vi "random number array generator.vi"() -> ()   [LabVIEW 2015]
panel:
  out "Random Numbers":dbl[](graph)
  in  "Iterations":i32
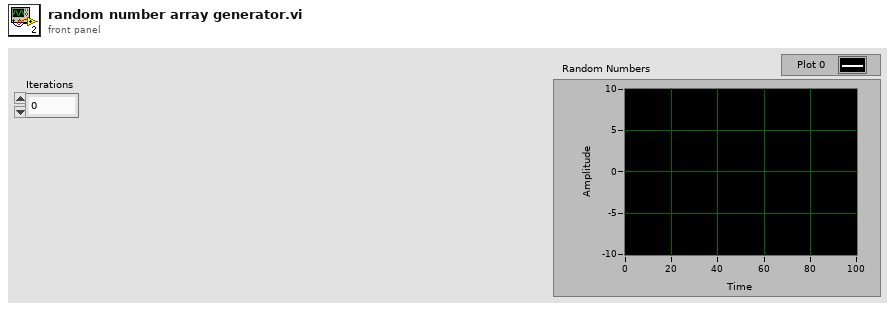
[diagram p1: front panel]
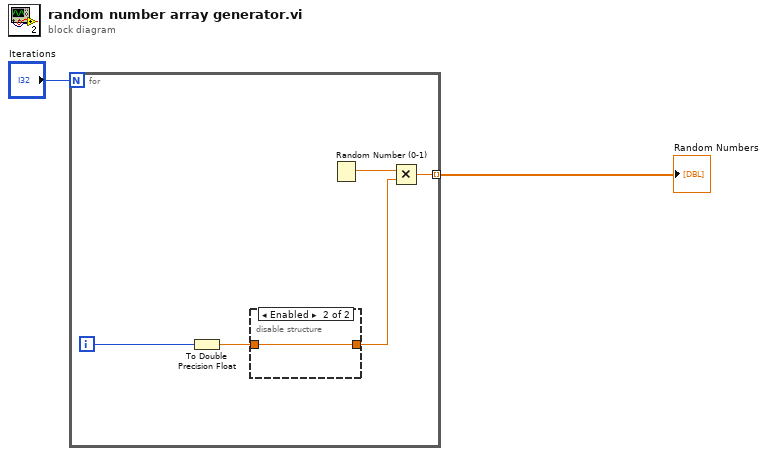
[diagram p0: block diagram]
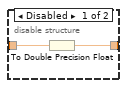
[diagram p2: hidden frame]
diagram:
  n1 = for {
    N: "Iterations" -> [_]
    tunnel: [w6] -> w1 mode=indexing
    i -> [w5]
    n2 = To Double Precision Float(number=w5) -> (double precision float=w4:dbl)
    n3 = disable-structure shown="Enabled" {
      disable-tunnel: w4 -> [w9 w10]
      disable-tunnel: [w8 w10] -> w3
      frame Disabled {
        n4 = To Double Precision Float(number=w9) -> (double precision float=w8:dbl)
      }
      frame Enabled {
      }
    }
    n5 = Random Number (0-1)() -> (number: 0 to 1=w7:dbl)
    n6 = Multiply(x=w7, y=w3) -> (x*y=w6:dbl)
  }
  "Random Numbers" <- w1
